vi "Parallel Channels Problem.vi"() -> ()   [LabVIEW 2023]
doc: "This example demonstrates the issues that arise when you include more than one communication channel between parallel while loops. Although some such architectures are safe, most lead to race conditions and deadlocks in code. In general, you want to avoid having mulitple communications channels, whether you are using LabVIEW \"channels\" or any other refnum/variable."
uses:
  <extravilib>/ChannelInstances/Tag-bool/Read With Abort.vi
  <extravilib>/ChannelInstances/Stream-i32/Read With Abort.vi
  <extravilib>/ChannelInstances/Tag-bool/Write With Abort.vi
  <extravilib>/ChannelInstances/Stream-i32/Write With Abort.vi
  <extravilib>/ChannelInstances/Stream-i32/EndpointRead.vi
  <extravilib>/ChannelInstances/Stream-i32/Endpoint.vi
  <extravilib>/ChannelInstances/Stream-i32/Instantiate.vi
  <extravilib>/ChannelInstances/Stream-i32/)Channel.vi
  <resource>/ChannelSupport/_ChannelSupport/WaitIfNeeded.vi
  <extravilib>/ChannelInstances/Tag-bool/Instantiate.vi
  <extravilib>/ChannelInstances/Tag-bool/EndpointRead.vi
  <extravilib>/ChannelInstances/Tag-bool/Endpoint.vi
  <extravilib>/ChannelInstances/Tag-bool.lvlib
  <extravilib>/ChannelInstances/Stream-i32.lvlib
panel:
  out "Consumed A":i32(graph)
  out "Consumed C":i32(graph)
  out "Produced C":i32(graph)
  in  "Stop Producer C":bool
  out "Consumed B":i32(graph)
  out "Produced B":i32(graph)
  in  "Stop Producer B":bool
  out "Produced A":i32(graph)
  in  "Stop Producer A":bool
  # "Overview: Demonstrates the problems that can arise when multiple communications systems are used between the same two loops. This applies to any communication system -- channels, refnums, variables, action engines, etc. -- but we can graphically demonstrate the issue with channels.\n\nInstructions:\n1. Run the VI. All three systems (A, B, & C) will start running.\n2. Press the Stop button for system A. It may or may not stop.\n3. Press the Stop buttons for B and C. They definitely will stop. \n4. If A did not stop, hit the Abort button for this VI. See the block diagram for details about why implementation A is unreliable.\n\nIf A did stop, run the VI a few more times. You may eventually get it to hang. On the other hand, you might be unlucky enough that this deadlock won't bite you at all until you put it on your production system. Race conditions are tricky like that."
  # "A. Unsafe"
  # "B. Safe - 2 Channels"
  # "C. Safe - 1 Channel"
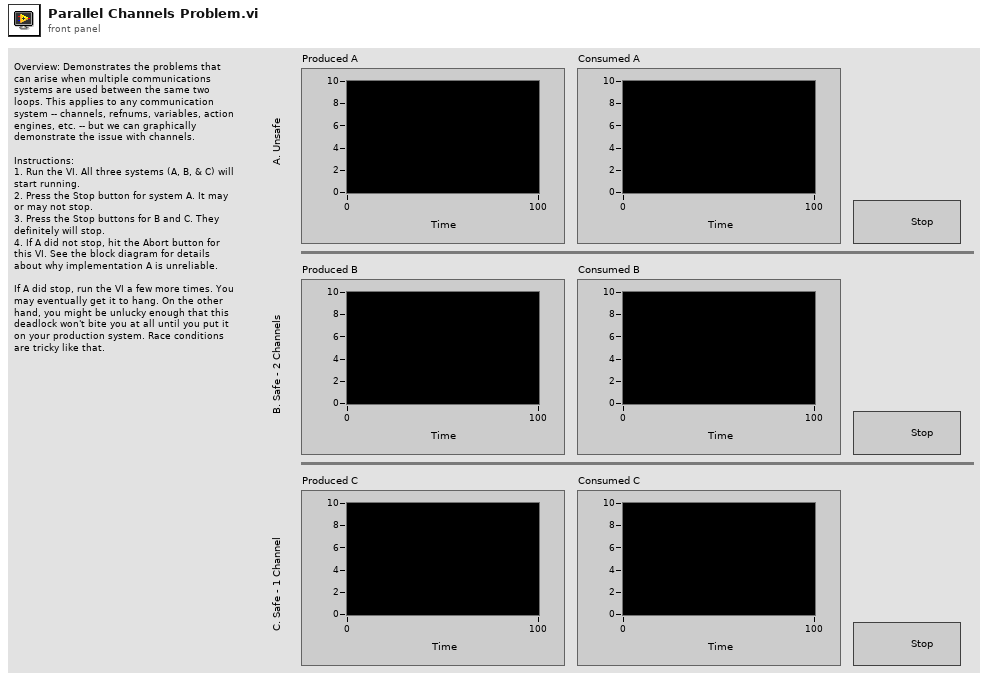
[diagram p1: front panel]
types:
  T1 = typedef "Stream-i32.lvlib/)Channel.ctl" = refnum<queue>
  T2 = typedef "Tag-bool.lvlib/))Channel.ctl" = refnum<queue>
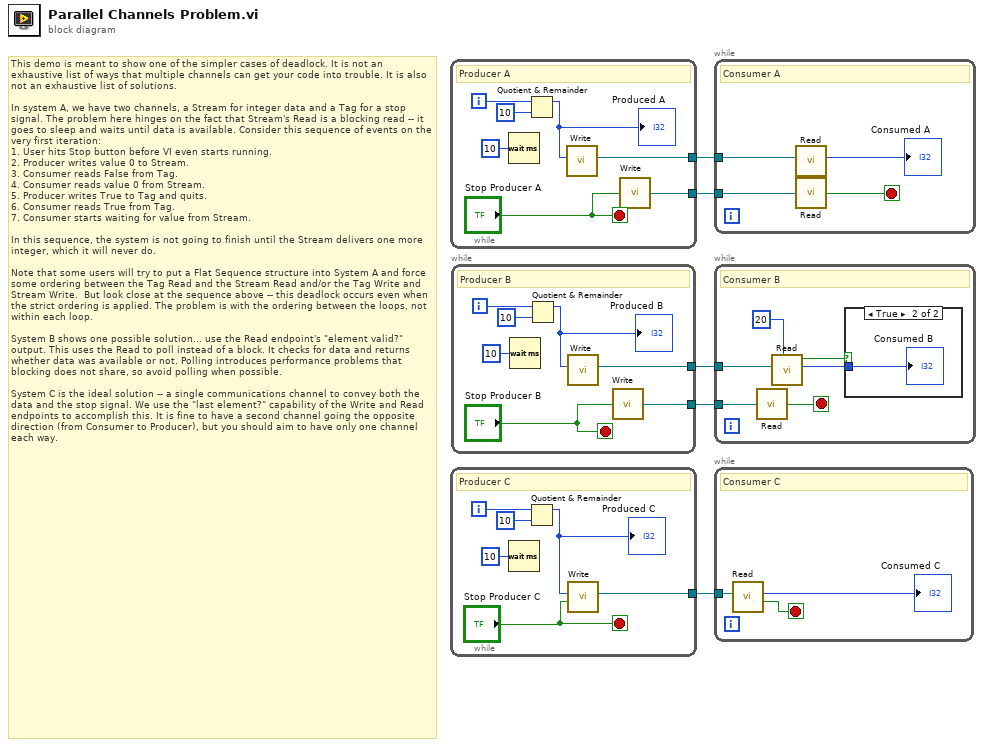
[diagram p0: block diagram]
diagram:
  # "This demo is meant to show one of the simpler cases of deadlock. It is not an exhaustive list of ways that multiple channels can get your code into trouble. It is also not an exhaustive list of solutions.\n\nIn system A, we have two channels, a Stream for integer data and a Tag for a stop signal. The problem here hinges on the fact that Stream's Read is a blocking read -- it goes to sleep and waits until data is available. Consider this sequence of events on the very first iteration:\n1. User hits Stop button before VI even starts running.\n2. Producer writes value 0 to Stream.\n3. Consumer reads False from Tag.\n4. Consumer reads value 0 from Stream.\n5. Producer writes True to Tag and quits.\n6. Consumer reads True from Tag.\n7. Consumer starts waiting for value from Stream.\n\nIn this sequence, the system is not going to finish until the Stream delivers one more integer, which it will never do.\n\nNote that some users will try to put a Flat Sequence structure into System A and force some ordering between the Tag Read and the Stream Read and/or the Tag Write and Stream Write.  But look close at the sequence above -- this deadlock occurs even when the strict ordering is applied. The problem is with the ordering between the loops, not within each loop.\n\nSystem B shows one possible solution... use the Read endpoint's \"element valid?\" output. This uses the Read to poll instead of a block. It checks for data and returns whether data was available or not. Polling introduces performance problems that blocking does not share, so avoid polling when possible.\n\nSystem C is the ideal solution -- a single communications channel to convey both the data and the stop signal. We use the \"last element?\" capability of the Write and Read endpoints to accomplish this. It is fine to have a second channel going the opposite direction (from Consumer to Producer), but you should aim to have only one channel each way."
  n1 = while {
    tunnel: [w9] -> w5
    tunnel: [w6] -> w4
    i -> [w11]
    stop <- "Stop Producer A" stop-if-true
    # "Producer A"
    n2 = Wait (ms)(milliseconds to wait=u32 10) -> ()  [unwired: 1 out]
    n3 = Quotient & Remainder(x=w11, y=10) -> (x-y*floor(x/y)=w10:i32)  [unwired: 1 out]
    "Produced A" <- w10
    n4 = call <extravilib>:"Write.vi"("element"=w10) -> ("channel"=w9:T1)  [unwired: 8 in, 2 out]
    n5 = call <extravilib>:"Write.vi"("element"="Stop Producer A") -> ("channel"=w6:T2)  [unwired: 1 out]
  }
  n6 = while {
    tunnel: [w16] -> w1
    i -> [w17]
    stop <- "Stop Producer C" stop-if-true
    # "Producer C"
    n7 = Wait (ms)(milliseconds to wait=u32 10) -> ()  [unwired: 1 out]
    n8 = Quotient & Remainder(x=w17, y=10) -> (x-y*floor(x/y)=w14:i32)  [unwired: 1 out]
    "Produced C" <- w14
    n9 = call <extravilib>:"Write.vi"("last element? (F)"="Stop Producer C", "element"=w14) -> ("channel"=w16:T1)  [unwired: 7 in, 2 out]
  }
  n10 = while {
    tunnel: [w23] -> w2
    tunnel: [w21] -> w3
    i -> [w24]
    stop <- "Stop Producer B" stop-if-true
    # "Producer B"
    n11 = Wait (ms)(milliseconds to wait=u32 10) -> ()  [unwired: 1 out]
    n12 = Quotient & Remainder(x=w24, y=10) -> (x-y*floor(x/y)=w19:i32)  [unwired: 1 out]
    "Produced B" <- w19
    n13 = call <extravilib>:"Write.vi"("element"=w19) -> ("channel"=w23:T1)  [unwired: 8 in, 2 out]
    n14 = call <extravilib>:"Write.vi"("element"="Stop Producer B") -> ("channel"=w21:T2)  [unwired: 1 out]
  }
  n15 = while {
    tunnel: w5 -> [w27]
    tunnel: w4 -> [w29]
    stop <- w28 stop-if-true
    # "Consumer A"
    n16 = call <extravilib>:"Read.vi"("channel"=w27) -> ("element"=→"Consumed A":i32)  [unwired: 6 in, 4 out]
    n17 = call <extravilib>:"Read.vi"("channel"=w29) -> ("element"=w28:bool)  [unwired: 1 in, 1 out]
  }
  n18 = while {
    tunnel: w2 -> [w33]
    tunnel: w3 -> [w35]
    stop <- w34 stop-if-true
    # "Consumer B"
    n19 = call <extravilib>:"Read.vi"("channel"=w35) -> ("element"=w34:bool)  [unwired: 1 in, 1 out]
    n20 = call <extravilib>:"Read.vi"("timeout in ms (-1)"=20 ("milliseconds to wait"), "channel"=w33) -> ("element"=w32:i32, "element valid?"=w31:bool)  [unwired: 5 in, 3 out]
    n21 = case shown="True" w31 {
      tunnel: w32 -> [_ w36]
      frame False {
      }
      frame True {
        "Consumed B" <- w36
      }
    }
  }
  n22 = while {
    tunnel: w1 -> [w39]
    stop <- w37 stop-if-true
    # "Consumer C"
    n23 = call <extravilib>:"Read.vi"("channel"=w39) -> ("last element?"=w37:bool, "element"=→"Consumed C":i32)  [unwired: 6 in, 3 out]
  }
